vi "Initialize.vi"(6 "Serial Flow Control (None)":u16(ring) items=["None", "XON/XOFF", "RTS/CTS", "XON/XOFF & RTS/CTS", "DTR/DSR", "XON/XOFF & DTR/DSR"], 7 "Serial Configuration":T1={"Baud Rate (9600)"=9600, "Parity (0: None)"=0, "Data Bits (8)"=8} {"Data Bits (8)" items=["7"=7, "8"=8]; "Parity (0: None)" items=["None", "Odd", "Even", "Mark", "Space"]; "Baud Rate (9600)" items=["300"=300, "600"=600, "1200"=1200, "2400"=2400, "4800"=4800, "9600"=9600]}, 8 "error in (no error)":errorcluster, 9 "Reset? (T: Yes)":bool=TRUE, 10 "ID Query? (T: Yes)":bool=TRUE, 11 "VISA resource name":refnum<visa-resource-name>) -> (0 "error out":errorcluster, 3 "VISA resource name out":refnum<visa-resource-name>)   [LabVIEW 2020, in "Agilent E363X Series.lvlib"]
doc: "Establishes communication with the instrument and optionally performs an instrument identification query and/or an instrument reset. It also places the instrument in a default state needed for other instrument driver operations. Therefore, call this VI before calling other instrument driver VIs for this instrument. Generally, you need to call the <B>Initialize VI</B> only once at the beginning of an application.\n\n<B>Notes:</B>\n<B>1. </B>When using the serial interface, the front panel buttons will be disabled unless the <B>local</B> button is pressed. Communicating over the serial interface can cause unexpected results and this is required as a precaution.\n\n<B>2. </B>Different instrument models supported by this instrument driver require a different <B>Serial Flow Control.</B>"
uses:
  Agilent E363X Series.lvlib
panel:
  # "(c) 2008 National Instruments.  ALL RIGHTS RESERVED."
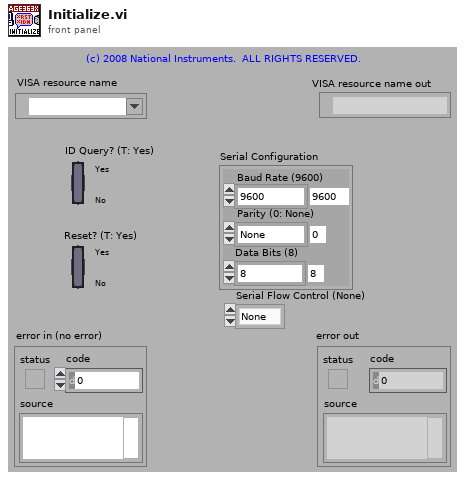
[diagram p1: front panel]
types:
  T1 = cluster{"Baud Rate (9600)":u32, "Parity (0: None)":u16, "Data Bits (8)":u16}
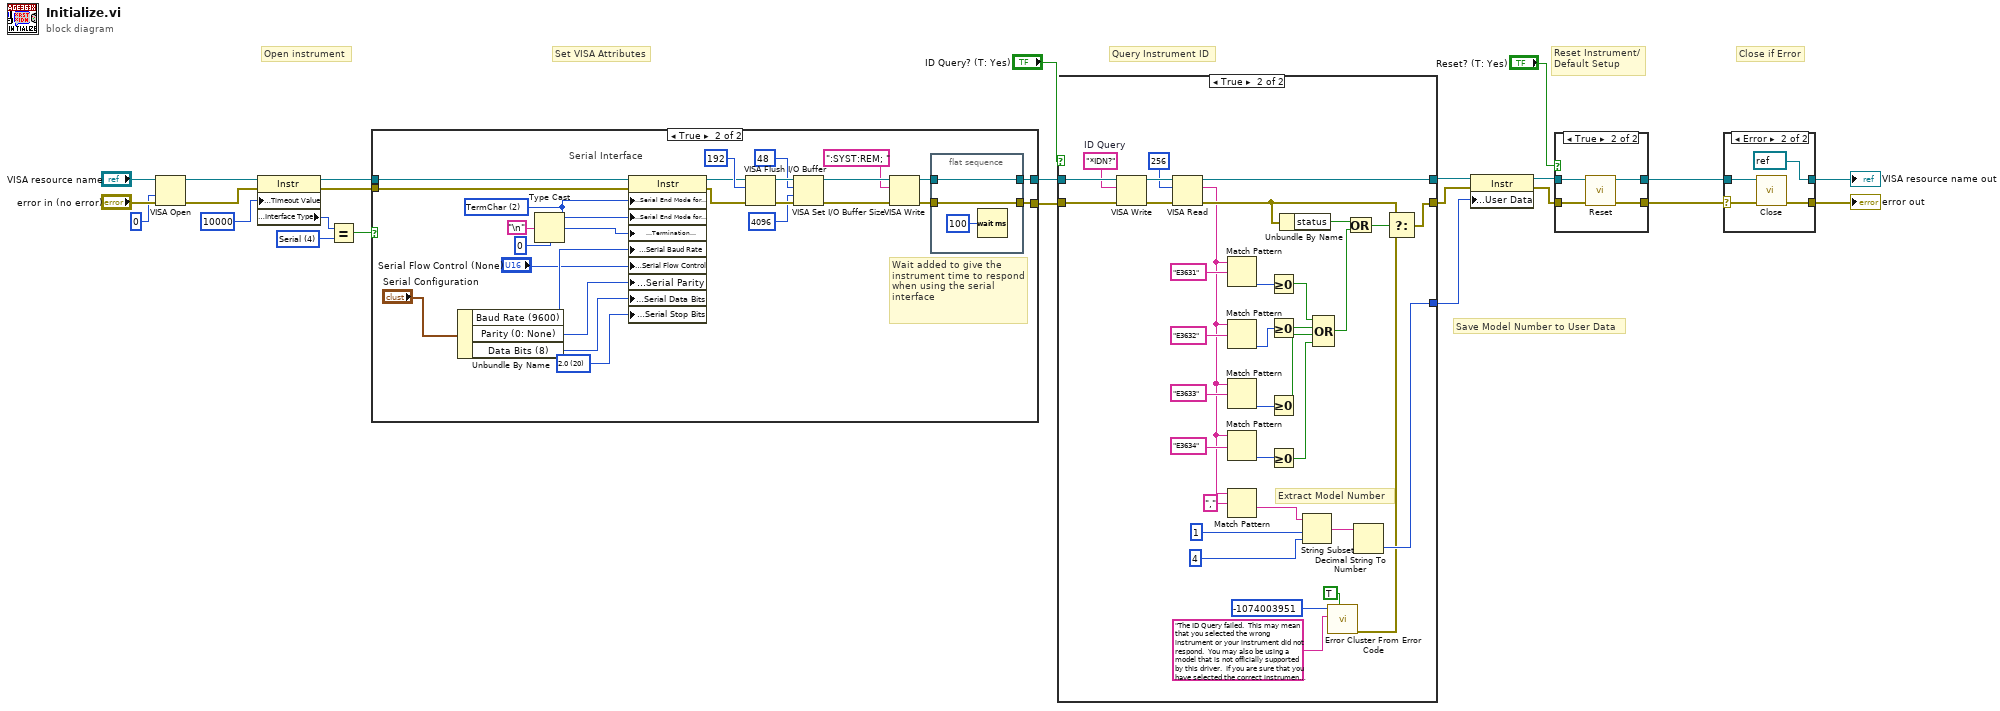
[diagram p0: block diagram]
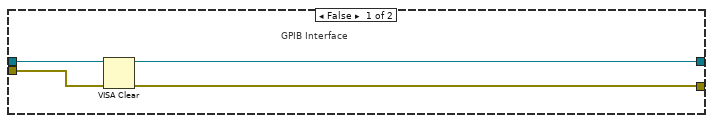
[diagram p2: hidden frame]
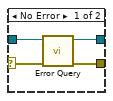
[diagram p3: hidden frame]
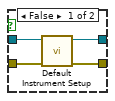
[diagram p4: hidden frame]
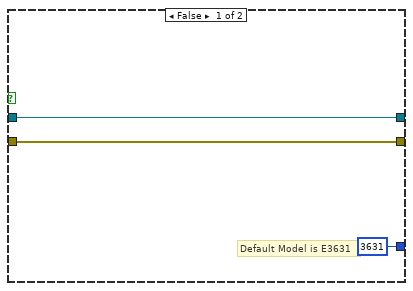
[diagram p5: hidden frame]
diagram:
  w13 = u16 4 items=["GPIB"=1, "VXI"=2, "GPIB-VXI"=3, "Serial"=4, "PXI"=5, "TCPIP"=6, "USB"=7] ("Interface Information:Interface Type")
  # "Save Model Number to User Data"
  # "Set VISA Attributes"
  # "Close if Error"
  # "Query Instrument ID"
  # "Reset Instrument/\nDefault Setup"
  # "Open instrument"
  n1 = VISA Open(access mode=u32 0, error in (no error)="error in (no error)", VISA resource name="VISA resource name") -> (VISA resource name=w2:refnum<visa-resource-name>, error out=w1:errorcluster)  [unwired: 2 in]
  n2 = property on="Property Node" class="Instr"(reference=w2, error in=w1, "General Settings:Timeout Value"=u32 10000) -> (reference out=w16:refnum<visa-resource-name>, error out=w15:errorcluster, "Interface Information:Interface Type"=w20:u16)
  n3 = Equal?(x=w20, y=w13) -> (x = y?=w14:bool)
  n4 = case shown="True" w14 {
    tunnel: [w25 w31] -> w18
    tunnel: [w27 w29] -> w17
    tunnel: w16 -> [w26 w45]
    tunnel: w15 -> [w28 w44]
    frame False {
      # "GPIB Interface"
      n5 = VISA Clear(VISA resource name=w26, error in (no error)=w28) -> (VISA resource name out=w25:refnum<visa-resource-name>, error out=w27:errorcluster)
    }
    frame True {
      w38 = u16 2 items=["None", "LastBit", "TermChar"] ("Serial Settings:Serial End Mode for Reads")
      w33 = u16 20 items=["1.0"=10, "1.5"=15, "2.0"=20] ("Serial Settings:Serial Stop Bits")
      # "Wait added to give the \ninstrument time to respond when using the serial interface"
      # "Serial Interface"
      n6 = Unbundle By Name("Serial Configuration") -> ("Baud Rate (9600)"=w37:u32, "Parity (0: None)"=w35:u16, "Data Bits (8)"=w34:u16)
      n7 = Type Cast(type=u8 0, x="\n" ("Line Feed Constant")) -> (*(type *) &x=w39:u8)
      n8 = property class="Instr"(reference=w45, error in=w44, "Serial Settings:Serial End Mode for Reads"=w38, "Serial Settings:Serial End Mode for Writes"=w38, "Message Based Settings:Termination Character"=w39, "Serial Settings:Serial Baud Rate"=w37, "Serial Settings:Serial Flow Control"="Serial Flow Control (None)", "Serial Settings:Serial Parity"=w35, "Serial Settings:Serial Data Bits"=w34, "Serial Settings:Serial Stop Bits"=w33) -> (reference out=w43:refnum<visa-resource-name>, error out=w42:errorcluster)
      n9 = VISA Flush I/O Buffer(VISA resource name=w43, mask (16)=u16 192, error in (no error)=w42) -> (VISA resource name out=w54:refnum<visa-resource-name>, error out=w53:errorcluster)
      n10 = VISA Set I/O Buffer Size(VISA resource name=w54, mask (16)=u16 48, size (4096)=u32 4096 ("size (0)"), error in (no error)=w53) -> (VISA resource name out=w47:refnum<visa-resource-name>, error out=w48:errorcluster)
      n11 = VISA Write(VISA resource name=w47, write buffer=":SYST:REM; ", error in (no error)=w48) -> (VISA resource name out=w32:refnum<visa-resource-name>, error out=w30:errorcluster)  [unwired: 1 out]
      n12 = flat-sequence {
        tunnel: w32 -> [w56]
        tunnel: [w56] -> w31
        tunnel: w30 -> [w55]
        tunnel: [w55] -> w29
        frame #0 {
          n13 = Wait (ms)(milliseconds to wait=u32 100) -> ()  [unwired: 1 out]
        }
      }
    }
  }
  n14 = case shown="True" "ID Query? (T: Yes)" {
    tunnel: [w59 w95] -> w6
    tunnel: [w60 w92] -> w5
    tunnel: w18 -> [w60 w93]
    tunnel: w17 -> [w59 w94]
    tunnel: [3631 ("offset past number") w65] -> w7
    frame False {
      # "Default Model is E3631"
    }
    frame True {
      w84 = "*IDN?"  # ID Query
      # "Extract Model Number"
      n15 = VISA Write(VISA resource name=w93, write buffer=w84, error in (no error)=w94) -> (VISA resource name out=w91:refnum<visa-resource-name>, error out=w89:errorcluster)  [unwired: 1 out]
      n16 = VISA Read(VISA resource name=w91, byte count=u32 256, error in (no error)=w89) -> (VISA resource name out=w92:refnum<visa-resource-name>, read buffer=w71:string, error out=w90:errorcluster)  [unwired: 1 out]
      n17 = Match Pattern(string=w71, regular expression="E3631") -> (offset past match=w80:i32)  [unwired: 1 in, 3 out]
      n18 = Match Pattern(string=w71, regular expression="E3632") -> (offset past match=w72:i32)  [unwired: 1 in, 3 out]
      n19 = Match Pattern(string=w71, regular expression="E3633") -> (offset past match=w73:i32)  [unwired: 1 in, 3 out]
      n20 = Match Pattern(string=w71, regular expression="E3634") -> (offset past match=w74:i32)  [unwired: 1 in, 3 out]
      n21 = Match Pattern(string=w71, regular expression=",") -> (after substring=w67:string)  [unwired: 1 in, 3 out]
      n22 = Greater Or Equal To 0?(x=w80) -> (x >= 0?=w78:bool)
      n23 = Greater Or Equal To 0?(x=w72) -> (x >= 0?=w77:bool)
      n24 = Greater Or Equal To 0?(x=w73) -> (x >= 0?=w76:bool)
      n25 = Greater Or Equal To 0?(x=w74) -> (x >= 0?=w75:bool)
      n26 = Unbundle By Name(w90) -> ("status"=w87:bool)
      n27 = String Subset(string=w67, offset (0)=1, length (rest)=4 ("length (rest)")) -> (substring=w66:string)
      n28 = Compound Arithmetic op=OR(w78, w77, w76, w75) -> (w79:bool)
      n29 = call <vilib>:"Error Cluster From Error Code.vi"("show call chain? (False)"=TRUE, "error message (\"\")"="The ID Query failed.  This may mean that you selected the wrong instrument or your instrument did not respond.  You may also be using a model that is not officially supported by this driver.  If you are sure that you have selected the correct instrument and it is responding, try disabling the ID Query." ("Source (VI Name)"), "error code (0)"=-1074003951 ("Code")) -> ("error out"=w61:errorcluster)  [unwired: 6 in]
      n30 = Or(x=w87, y=w79) -> (x .or. y?=w88:bool)
      n31 = Decimal String To Number(string=w66) -> (number=w65:i32)  [unwired: 2 in, 1 out]
      n32 = Select(t=w90, s=w88, f=w61) -> (s? t:f=w95:errorcluster)
    }
  }
  n33 = property on="Property Node" class="Instr"(reference=w5, error in=w6, "General Settings:User Data"=w7) -> (reference out=w4:refnum<visa-resource-name>, error out=w3:errorcluster)
  n34 = case shown="True" "Reset? (T: Yes)" {
    tunnel: w3 -> [w98 w100]
    tunnel: [w97 w103] -> w8
    tunnel: w4 -> [w99 w101]
    tunnel: [w96 w102] -> w9
    frame False {
      n35 = call "Default Instrument Setup.vi"("error in (no error)"=w98, "VISA resource name"=w99) -> ("error out"=w97:errorcluster, "VISA resource name out"=w96:refnum<visa-resource-name>)  [unwired: 8 in]
    }
    frame True {
      n36 = call "Reset.vi"("error in (no error)"=w100, "VISA resource name"=w101) -> ("error out"=w103:errorcluster, "VISA resource name out"=w102:refnum<visa-resource-name>)  [unwired: 8 in]
    }
  }
  n37 = case shown="Error" w8 {
    selector: w8 -> [w105 w109]
    tunnel: w9 -> [w104 w110]
    tunnel: [w107 refnum<visa-resource-name> refnum ("VISA resource name out")] -> w11
    tunnel: [w106 w111] -> w10
    frame No Error {
      n38 = call "Error Query.vi"("error in (no error)"=w105, "VISA resource name"=w104) -> ("error out"=w106:errorcluster, "VISA resource name out"=w107:refnum<visa-resource-name>)  [unwired: 6 in, 2 out]
    }
    frame Error {
      n39 = call "Close.vi"("error in (no error)"=w109, "VISA resource name"=w110) -> ("error out"=w111:errorcluster)  [unwired: 9 in]
    }
  }
  "VISA resource name out" <- w11
  "error out" <- w10
